vi "writeToXML.vi"(8 "error in (no error)":errorcluster, 10 "ClassLabel":string, 11 "TCSDebug in":refnum<class "TCSDebug.lvclass">) -> (0 "error out":errorcluster, 2 "XML out":string, 3 "TCSDebug out":refnum<class "TCSDebug.lvclass">)   [LabVIEW 2022 SP3, in "TCSDataDefinitions.lvlib" / "TCSCommand.lvlib" / "TCSDebug.lvclass"]
uses:
  TCSDebug.lvclass
  TCSDebug.lvclass/TCSDebug.ctl
  TCSTcsCommand/TCSTcsCommand.lvclass
  <userlib>/Common/XML/XMLGenerator/XMLGenerator.lvclass
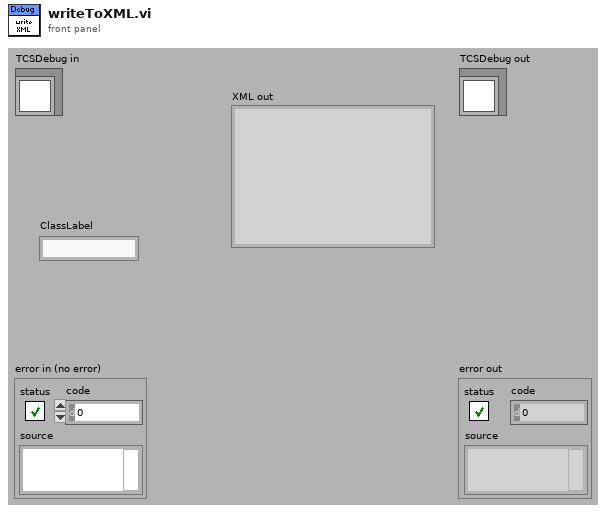
[diagram p1: front panel]
types:
  T1 = typedef "TCSDataDefinitions.lvlib/TCSCommand.lvlib/TCSDebuLevelTypes.ctl" = enum16{"0", "1", "2", "3", "4", "5", "6", "7", "8", "9", "10"}
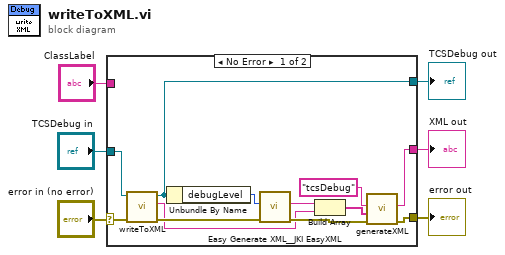
[diagram p0: block diagram]
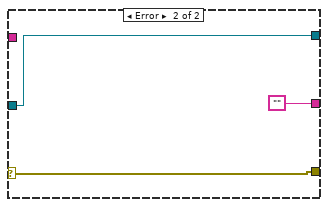
[diagram p2: hidden frame]
diagram:
  n1 = case shown="No Error" "error in (no error)" {
    selector: "error in (no error)" -> [w10 w21]
    tunnel: [w8 w21] -> w5
    tunnel: [w12 w20] -> w3
    tunnel: "TCSDebug in" -> [w13 w20]
    tunnel: "ClassLabel" -> [_ _]
    tunnel: [w14 ""] -> w1
    frame No Error {
      n2 = call-parent "writeToXML.vi"("error in (no error)"=w10, "TCSTcsCommand in"=w13) -> ("error out"=w9:errorcluster, "XML out"=w7:string, "TCSTcsCommand out"=w12:refnum<class "TCSDebug.lvclass">)  [unwired: 7 in]
      n3 = Unbundle By Name(w12) -> ("debugLevel"=w18:T1)
      n4 = call <vilib>:"Easy Generate XML__JKI EasyXML.vi"("error in (no error)"=w9, "LabVIEW Data"=w18) -> ("error out"=w15:errorcluster, "XML String"=w16:string)  [unwired: 8 in]
      n5 = Build Array(w16, w7) -> (w17:string[])
      n6 = call <userlib>:"generateXML.vi"("error in"=w15, "childrenXML"=w17, "elementName"="tcsDebug" ("Class Label")) -> ("error out"=w8:errorcluster, "XML out"=w14:string)  [unwired: 6 in, 1 out]
    }
    frame Error {
    }
  }
  "error out" <- w5
  "TCSDebug out" <- w3
  "XML out" <- w1
